vi "Fishing Continuous OCR.vi"() -> ()   [LabVIEW 2019]
doc: "This VI captures the region of the screen and displays it on the front panel continuously.\nCan be used to develop remote desktop applications."
uses:
  <vilib>/Utility/miscctls.llb/LVBoundsTypeDef.ctl
  System.Drawing
  <vilib>/Instr/_visa.llb/VISA Configure Serial Port (Instr).vi
  <vilib>/Utility/inputDevices.llb/mouseAcquire.vi
  <vilib>/Utility/inputDevices.llb/closeMouse.vi
  <vilib>/wsapi/NI_WebServices.lvlib
panel:
  out "Max Occ":string
  out "max index(es)":i32
  in  "Reset Array":bool
  out "Count A":dbl[](array[numeric])
  out "String A":string[](array[string])
  out "Init Error":errorcluster
  out "Length":i32
  out "Tx":string
  in  "String Cont":string
  out "Return Count":u32
  out "COM Status":bool
  in  "MC COM Port":refnum<visa-resource-name>="COM5"
  out "Processed Image":T1(plugin-control)
  out "Filtered String Output":string
  in  "Delay (ms)":i32=100
  in  "Error In":errorcluster
  out "Mouse y":dbl
  out "Mouse x":dbl
  in  "Height (px)":i32=100
  in  "Width (px)":i32=600
  out "Screen Capture":picture
  in  "stop":bool
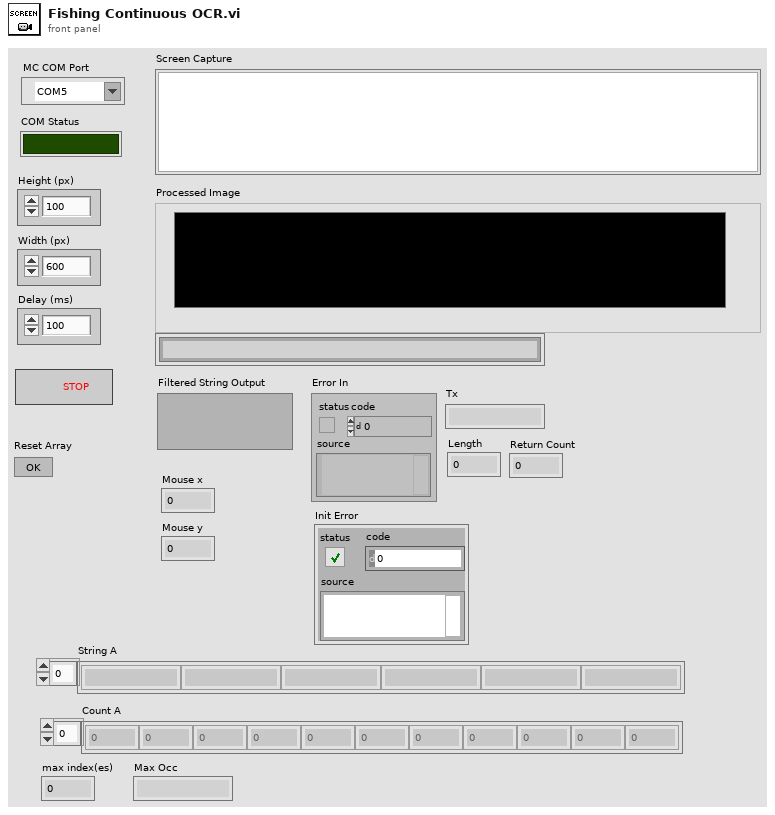
[diagram p1: front panel]
types:
  T1 = typedef "IMAQ Image.ctl" = refnum<image>
  T2 = typedef "LVBoundsTypeDef.ctl" = cluster{"Width":u32, "Height":u32}
  T3 = typedef "Image Type" = u32
  T4 = cluster{"Horizontal":i32, "Vertical":i32, "Scrolling":i32}
  T5 = typedef "imagedata.ctl" = cluster{"image type":i32, "image depth":i32, "image":u8[], "mask":u8[], "colors":u32[], "Rectangle":cluster{"left":i16, "top":i16, "right":i16, "bottom":i16}}
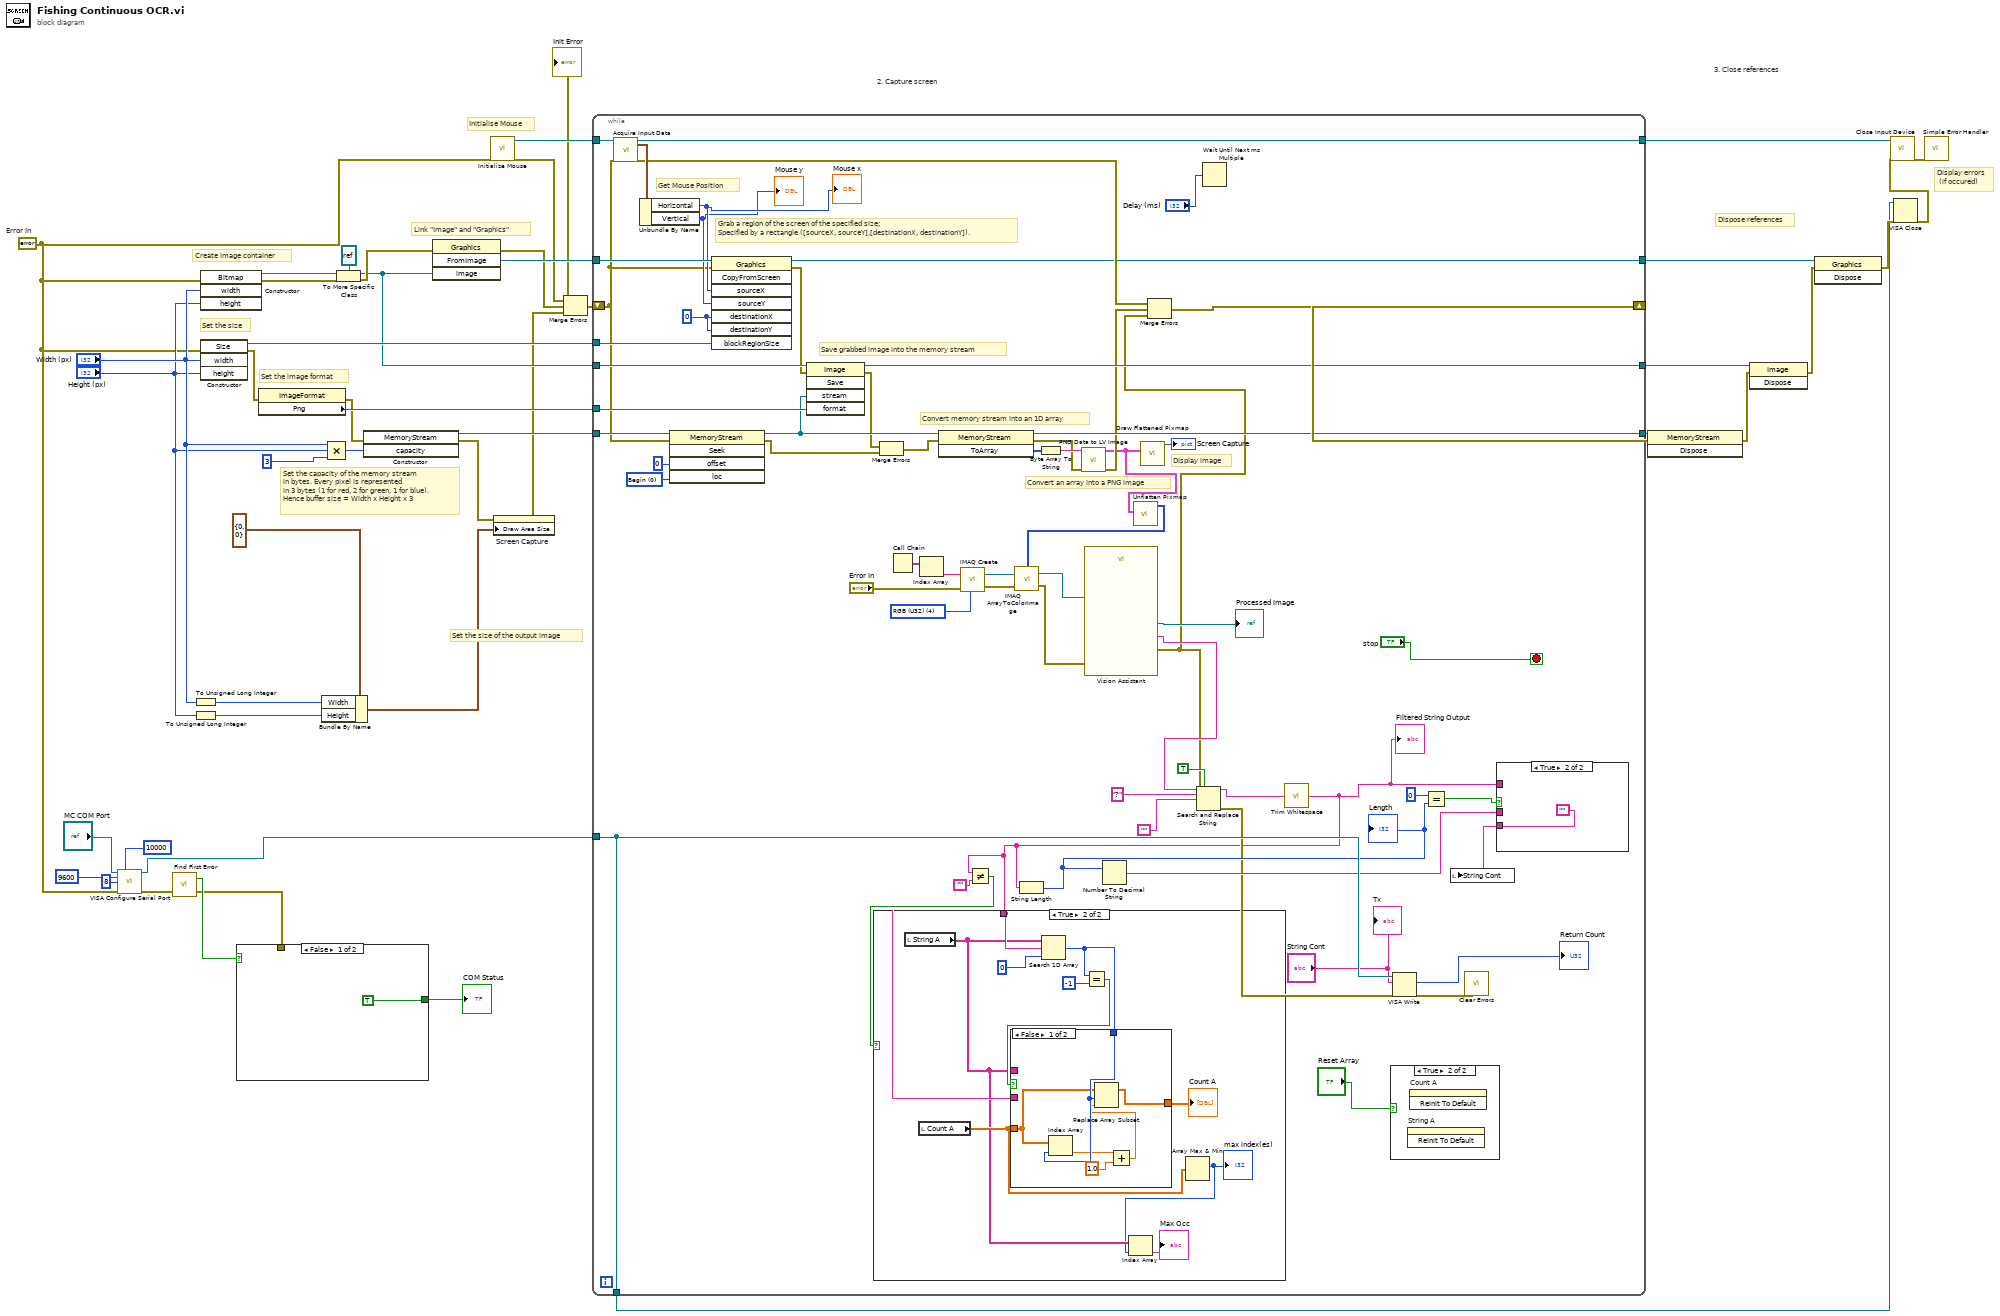
[diagram p0: block diagram]
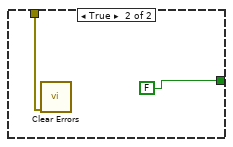
[diagram p2: hidden frame]
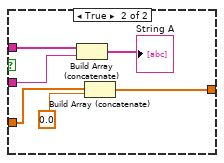
[diagram p4: hidden frame]
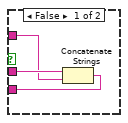
[diagram p6: hidden frame]
diagram:
  w12 = errorcluster {"status"=FALSE, "code"=0, "source"=""}  # Error In
  # "Link \"Image\" and \"Graphics\""
  # "Set the size"
  # "Create image container"
  # "3. Close references"
  # "2. Capture screen"
  # "Display errors\n (if occured)"
  # "Dispose references"
  # "Set the image format"
  # "Set the size of the output image"
  # "Set the capacity of the memory stream\nin bytes. Every pixel is represented\nin 3 bytes (1 for red, 2 for green, 1 for blue).\nHence buffer size = Width x Height x 3"
  # "Initialise Mouse"
  n1 = call-poly "VISA Configure Serial Port"("VISA resource name"="MC COM Port", "timeout (10sec)"=u32 10000, "baud rate (9600)"=u32 9600, "data bits (8)"=u16 8, "error in (no error)"=w12) -> ("VISA resource name out"=w1:refnum<visa-resource-name>, "error out"=w11:errorcluster)  [unwired: 9 in]
  n2 = call <vilib>:"Find First Error.vi"("error in (no error)"=w11) -> ("error out"=w8:errorcluster, "error?"=w10:bool)  [unwired: 3 in]
  n3 = To Unsigned Long Integer(number="Width (px)") -> (unsigned 32bit integer=w20:u32)
  n4 = To Unsigned Long Integer(number="Height (px)") -> (unsigned 32bit integer=w18:u32)
  n5 = constructor class="Bitmap"(error in=w12, "width"="Width (px)", "height"="Height (px)") -> (reference out=w40:refnum<k24>, error out=w43:errorcluster)  [unwired: 2 in, 3 out]
  n6 = constructor class="Size"(error in=w12, "width"="Width (px)", "height"="Height (px)") -> (reference out=w38:refnum<k24>, error out=w29:errorcluster)  [unwired: 2 in, 3 out]
  n7 = case shown="False" w10 {
    tunnel: [TRUE FALSE] -> w9
    tunnel: w8 -> [_ w48]
    frame False {
    }
    frame True {
      n8 = call <vilib>:"Clear Errors.vi"("error in (no error)"=w48) -> ()  [unwired: 5 in, 2 out]
    }
  }
  "COM Status" <- w9
  n9 = property class="ImageFormat"(error in=w29) -> (error out=w28:errorcluster, "Png"=w37:refnum<k24>)  [unwired: 1 in, 1 out]
  n10 = Bundle By Name(cluster=T2 {"Width"=0, "Height"=0} ("Draw Area Size"), "Width"=w20, "Height"=w18) -> (w24:T2)
  n11 = Compound Arithmetic op=MULTIPLY("Width (px)", "Height (px)", 3 ("value")) -> (w32:i32)
  n12 = To More Specific Class(target class=refnum<k24> refnum, reference=w40, error in=w43) -> (specific class reference=w31:refnum<k24>, error out=w44:errorcluster)
  n13 = constructor class="MemoryStream"(error in=w28, "capacity"=w32) -> (reference out=w34:refnum<k24>, error out=w23:errorcluster)  [unwired: 2 in, 2 out]
  n14 = invoke class="Graphics" method="FromImage"(error in=w44, "image"=w31) -> (error out=w27:errorcluster, "FromImage"=w41:refnum<k24>)  [unwired: 2 in, 2 out]
  n15 = call <vilib>:"Initialize Mouse.vi"("error in (no error)"=w12) -> ("error out"=w25:errorcluster, "device ID"=w46:refnum<k1>)  [unwired: 9 in]
  n16 = property on="Screen Capture" class="Pict"(error in=w23, "Draw Area Size"=w24) -> (error out=w22:errorcluster)  [unwired: 1 in, 1 out]
  n17 = Merge Errors(w25, w27, w22) -> (w26:errorcluster)
  "Init Error" <- w26
  n18 = while {
    tunnel: w46 -> [w111]
    tunnel: [w109] -> w45
    tunnel: w41 -> [w108]
    tunnel: [w105] -> w39
    tunnel: w38 -> [w104]
    tunnel: w37 -> [w103]
    tunnel: [w102] -> w36
    tunnel: w34 -> [w101]
    tunnel: w31 -> [w95]
    shift-right: [w87] -> w14
    shift-left: w26 -> [w65]
    tunnel: [w86] -> w17
    tunnel: w1 -> [w64]
    tunnel: [w64] -> w5
    stop <- "stop" stop-if-true
    w78 = T3 4 items=["Grayscale (U8)", "Grayscale (I16)", "Grayscale (SGL)", "Complex (CSG)", "RGB (U32)", "HSL (U32)", "RGB (U64)", "Grayscale (U16)"] ("Image Type")
    w96 = 0 ("destinationX")
    w99 = 0 items=["Begin", "Current", "End"] ("loc")
    # "Display image"
    # "Convert an array into a PNG image"
    # "Convert memory stream into an 1D array"
    # "Save grabbed image into the memory stream"
    # "Grab a region of the screen of the specified size;\nSpecified by a rectangle ([sourceX, sourceY],[destinationX, destinationY])."
    # "Get Mouse Position"
    n19 = call-poly <vilib>:"Acquire Input Data.vi"("device ID"=w111, "error in (no error)"=w65) -> ("device ID"=w109:refnum<k1>, "axis info"=w110:T4, "error out"=w89:errorcluster)  [unwired: 14 in, 1 out]
    n20 = Unbundle By Name(w110) -> ("Horizontal"=w85:i32, "Vertical"=w84:i32)
    "Mouse x" <- w85
    "Mouse y" <- w84
    n21 = invoke class="MemoryStream" method="Seek"(reference=w101, error in=w65, "offset"=i64 0, "loc"=w99) -> (reference out=w97:refnum<k24>, error out=w92:errorcluster)  [unwired: 1 in, 3 out]
    n22 = invoke class="Graphics" method="CopyFromScreen"(reference=w108, error in=w65, "sourceX"=w85, "sourceY"=w84, "destinationX"=w96, "destinationY"=w96, "blockRegionSize"=w104) -> (reference out=w86:refnum<k24>, error out=w90:errorcluster)  [unwired: 1 in, 6 out]
    n23 = invoke class="Image" method="Save"(reference=w95, error in=w90, "stream"=w97, "format"=w103) -> (reference out=w102:refnum<k24>, error out=w93:errorcluster)  [unwired: 1 in, 3 out]
    n24 = Merge Errors(w93, w92) -> (w91:errorcluster)
    n25 = Call Chain() -> (call chain=w80:string[])
    n26 = Index Array(array=w80) -> (element=w81:string)  [unwired: 1 in]
    n27 = invoke class="MemoryStream" method="ToArray"(reference=w97, error in=w91) -> (reference out=w105:refnum<k24>, error out=w94:errorcluster, "ToArray"=w107:u8[])  [unwired: 1 in]
    n28 = call "IMAQ Create"("Image Name"=w81, "Image Type"=w78, "error in (no error)"="Error In") -> ("New Image"=w77:T1, "error out"=w76:errorcluster)  [unwired: 1 in, 1 out]
    n29 = Byte Array To String(unsigned byte array=w107) -> (string=w106:string)
    n30 = call <vilib>:"PNG Data to LV Image.vi"("error in (no error)"=w94, "png data"=w106) -> ("error out"=w88:errorcluster, "image data"=w83:T5)  [unwired: 8 in]
    n31 = call <vilib>:"Unflatten Pixmap.vi"("image data"=w83) -> ("24-bit pixmap"=w82:u32[][])  [unwired: 4 in, 6 out]
    n32 = call "IMAQ ArrayToColorImage"("Image Pixels (U32)"=w82, "Image"=w77, "error in (no error)"=w76) -> ("Image Out"=w74:T1, "error out"=w75:errorcluster)  [unwired: 2 in]
    n33 = call "Vision Assistant"("Image In"=w74, "error in"=w75) -> ("Image Out"=→"Processed Image":T1, "String (OCR/OCV 2)"=w69:string, "error out"=w58:errorcluster)  [unwired: 23 in]
    n34 = call <vilib>:"Draw Flattened Pixmap.vi"("image data"=w83) -> ("new picture"=→"Screen Capture":picture)  [unwired: 8 in]
    n35 = Merge Errors(w89, w88, w58) -> (w87:errorcluster)
    n36 = Search and Replace String(replace all?=TRUE ("replace all? (F)"), input string=w69, search string="?", replace string="", error in=w58) -> (result string=w68:string, error out=w55:errorcluster)  [unwired: 3 in, 2 out]
    n37 = Wait Until Next ms Multiple(millisecond multiple="Delay (ms)") -> ()  [unwired: 1 out]
    n38 = call <vilib>:"Trim Whitespace.vi"("string"=w68) -> ("trimmed string"=w51:string)  [unwired: 1 in]
    "Filtered String Output" <- w51
    n39 = Not Equal?(x=w51, y="") -> (x != y?=w50:bool)
    n40 = case shown="True" w50 {
      tunnel: w51 -> [_ w116]
      frame False {
      }
      frame True {
        n41 = local read "String A"() -> (w114:string[])
        n42 = local read "Count A"() -> (w115:dbl[])
        n43 = Search 1D Array(1D array=w114, element=w116, start index (0)=0) -> (index of element=w118:i32)
        n44 = Equal?(x=w118, y=-1) -> (x = y?=w119:bool)
        n45 = case shown="False" w119 {
          tunnel: w114 -> [_ w133]
          tunnel: w116 -> [_ w132]
          tunnel: w118 -> [w127 _]
          tunnel: w115 -> [w123 w129]
          tunnel: [w122 w130] -> w117
          frame False {
            n46 = Index Array(array=w123, index=w127) -> (element=w125:dbl)
            n47 = Add(x=w125, y=1.0) -> (x+y=w124:dbl)
            n48 = Replace Array Subset(array=w123, new element=w124, index=w127) -> (w122:dbl[])
          }
          frame True {
            n49 = Build Array (concatenate)(w133, w132) -> (→"String A":string[])
            n50 = Build Array (concatenate)(w129, 0.0 ("new element/subarray")) -> (w130:dbl[])
          }
        }
        "Count A" <- w117
        n51 = Array Max & Min(array=w115) -> (max index (indices)=w113:i32)  [unwired: 3 out]
        "max index(es)" <- w113
        n52 = Index Array(array=w114, index=w113) -> (element=→"Max Occ":string)
      }
    }
    n53 = String Length(string=w51) -> (length=w62:i32)
    "Length" <- w62
    n54 = Number To Decimal String(number=w62) -> (decimal integer string=w60:string)  [unwired: 1 in]
    n55 = case shown="True" "Reset Array" {
      frame False {
      }
      frame True {
        n56 = invoke on="String A" class="Arr (strict)" method="Reinit To Default"() -> ()  [unwired: 3 in, 3 out]
        n57 = invoke on="Count A" class="Arr (strict)" method="Reinit To Default"() -> ()  [unwired: 3 in, 3 out]
      }
    }
    n58 = VISA Write(VISA resource name=w64, write buffer="String Cont", error in (no error)=w55) -> (return count=→"Return Count":u32, error out=w54:errorcluster)  [unwired: 1 out]
    n59 = Equal?(x=0, y=w62) -> (x = y?=w63:bool)
    n60 = call <vilib>:"Clear Errors.vi"("error in (no error)"=w54) -> ()  [unwired: 5 in, 2 out]
    n61 = case shown="True" w63 {
      tunnel: w60 -> [w136 _]
      tunnel: w51 -> [w135 _]
      tunnel: [w134 ""] -> w59
      frame False {
        n62 = Concatenate Strings(w136, w135) -> (w134:string)
      }
      frame True {
      }
    }
    n63 = local write "String Cont"(w59) -> ()
    "Tx" <- "String Cont"
  }
  n64 = invoke class="MemoryStream" method="Dispose"(reference=w39, error in=w14) -> (error out=w35:errorcluster)  [unwired: 1 in, 2 out]
  n65 = invoke class="Image" method="Dispose"(reference=w36, error in=w35) -> (error out=w16:errorcluster)  [unwired: 1 in, 2 out]
  n66 = invoke class="Graphics" method="Dispose"(reference=w17, error in=w16) -> (error out=w7:errorcluster)  [unwired: 1 in, 2 out]
  n67 = VISA Close(VISA resource name=w5, error in (no error)=w7) -> (error out=w6:errorcluster)
  n68 = call-poly <vilib>:"Close Input Device.vi"("error in (no error)"=w6, "device ID"=w45) -> ("error out"=w15:errorcluster)  [unwired: 8 in]
  n69 = call <vilib>:"Simple Error Handler.vi"("error in (no error)"=w15) -> ()  [unwired: 4 in, 5 out]
